vi "creat_user_event.vi"(8 "error in (no error)":errorcluster) -> (0 "error out":errorcluster, 3 "machine status":refnum<user-event>)   [LabVIEW 2013]
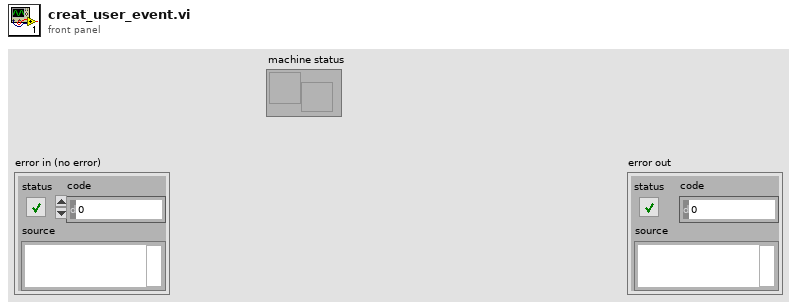
[diagram p1: front panel]
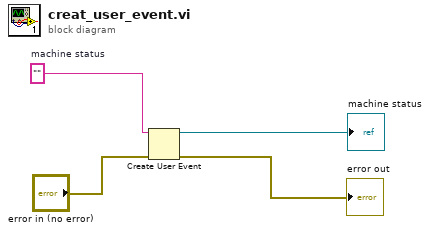
[diagram p0: block diagram]
diagram:
  w4 = ""  # machine status
  n1 = Create User Event(user event datatype=w4, error in="error in (no error)") -> (user event=→"machine status":refnum<user-event>, error out=→"error out":errorcluster)
